vi "继保软压板转.vi"(1 "软压板Rin":bool[](array[boolean])=[FALSE, FALSE, FALSE, FALSE, FALSE, FALSE, FALSE, FALSE, FALSE, FALSE, FALSE, FALSE] caption="软压板R") -> (0 "软压板Rout":T1 caption="继保遥信")   [LabVIEW 2015]
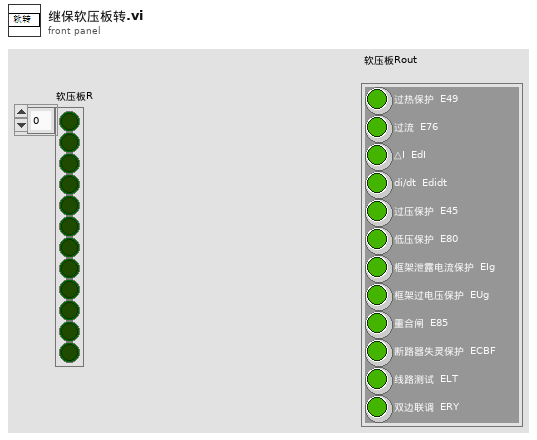
[diagram p1: front panel]
types:
  T1 = cluster{"过热保护  E49":bool, "过流  E76":bool, "△I  EdI":bool, "di/dt  Edidt":bool, "过压保护  E45":bool, "低压保护  E80":bool, "框架泄露电流保护  EIg":bool, "框架过电压保护  EUg":bool, "重合闸  E85":bool, "断路器失灵保护  ECBF":bool, "线路测试  ELT":bool, "双边联调  ERY":bool}
  T2 = cluster{"Boolean":bool, "Boolean":bool, "Boolean":bool, "Boolean":bool, "Boolean":bool, "Boolean":bool, "Boolean":bool, "Boolean":bool, "Boolean":bool, "Boolean":bool, "Boolean":bool, "Boolean":bool}
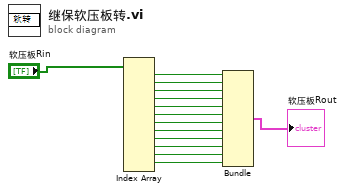
[diagram p0: block diagram]
diagram:
  n1 = Index Array(array="软压板Rin") -> (element #1=w13:bool, element #2=w12:bool, element #3=w11:bool, element #4=w10:bool, element #5=w9:bool, element #6=w8:bool, element #7=w7:bool, element #8=w6:bool, element #9=w5:bool, element #10=w4:bool, element #11=w3:bool, element #12=w2:bool)  [unwired: 12 in]
  n2 = Bundle("Boolean"=w13, "Boolean"=w12, "Boolean"=w11, "Boolean"=w10, "Boolean"=w9, "Boolean"=w8, "Boolean"=w7, "Boolean"=w6, "Boolean"=w5, "Boolean"=w4, "Boolean"=w3, "Boolean"=w2) -> (→"软压板Rout":T2)  [unwired: 1 in]
